vi "ECG_Monitor.vi"() -> ()   [LabVIEW 2011]
uses:
  <vilib>/Analysis/NI_AALBase.lvlib
  <vilib>/Analysis/3filter.llb/Butterworth Filter (DBL).vi
  <vilib>/Analysis/NI_AALPro.lvlib
  <vilib>/Analysis/2dsp.llb/Real FFT.vi
panel:
  out "Measured \nHeart Rate (bpm)":dbl
  in  "Set Threshold":i32(slide) scale=-600.0..600.0
  in  "start":bool
  in  "Save Data?":bool
  in  "High Cutoff Frequency (Hz)":i32
  in  "Filter Type":T1(ring)=enum."Band Pass"
  in  "Select Channel B":T2(ring)=enum."Zero"
  in  "Apply Filter?":bool
  in  "Low Cutoff Frequency (Hz)":i32=100
  out "Frequency Domain Signal":cluster{i32, dbl, "Power Spectrum":dbl[]}(graph)={0, 1.0, "Power Spectrum"=[]}
  out "Time Domain Signal":cluster{i32, dbl, dbl[]}(graph)={0, 1.0, []}
  in  "Select Channel A":enum16{"Channel 1", "Channel 2", "Channel 3"}(ring)
  out "Device Name":string="BioRadio 150"
  in  "Data Collection\nInterval (ms)":u32=1000
  in  "stop":bool
  out "DroppedPackets":u32
  out "BadPackets":u32
  out "GoodPackets":u32
  # "Transmission\nInformation"
  # "The signal observed below is given by (Channel A - Channel B)"
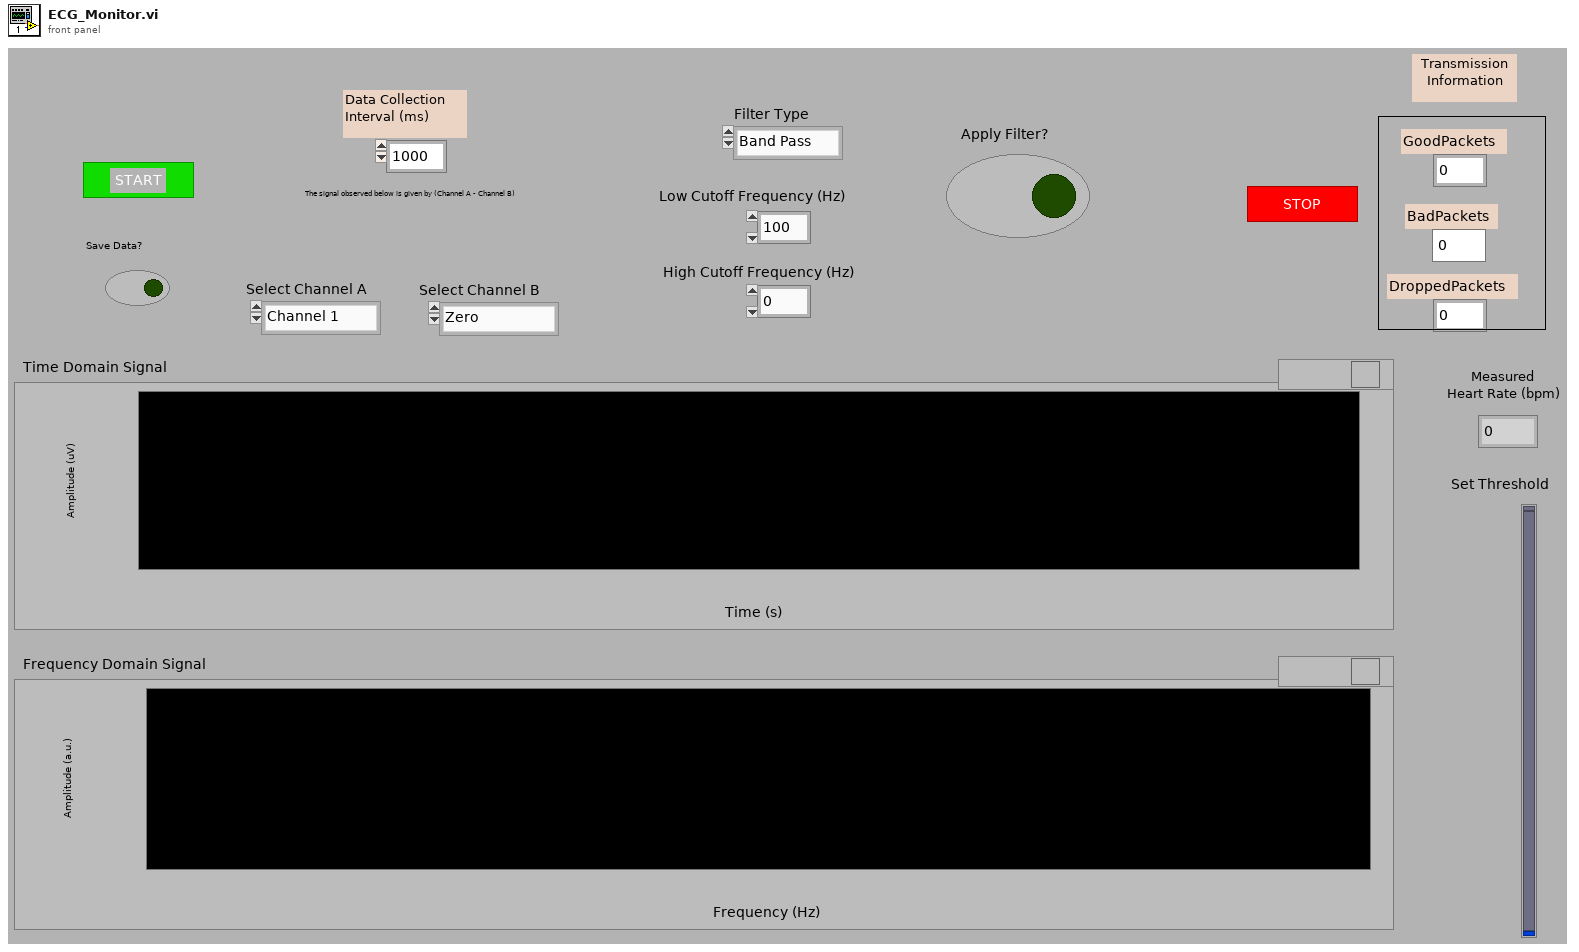
[diagram p1: front panel]
types:
  T1 = enum16{"Low Pass", "High Pass", "Band Pass", "Band Stop"}
  T2 = enum16{"Channel 1", "Channel 2", "Channel 3", "Zero"}
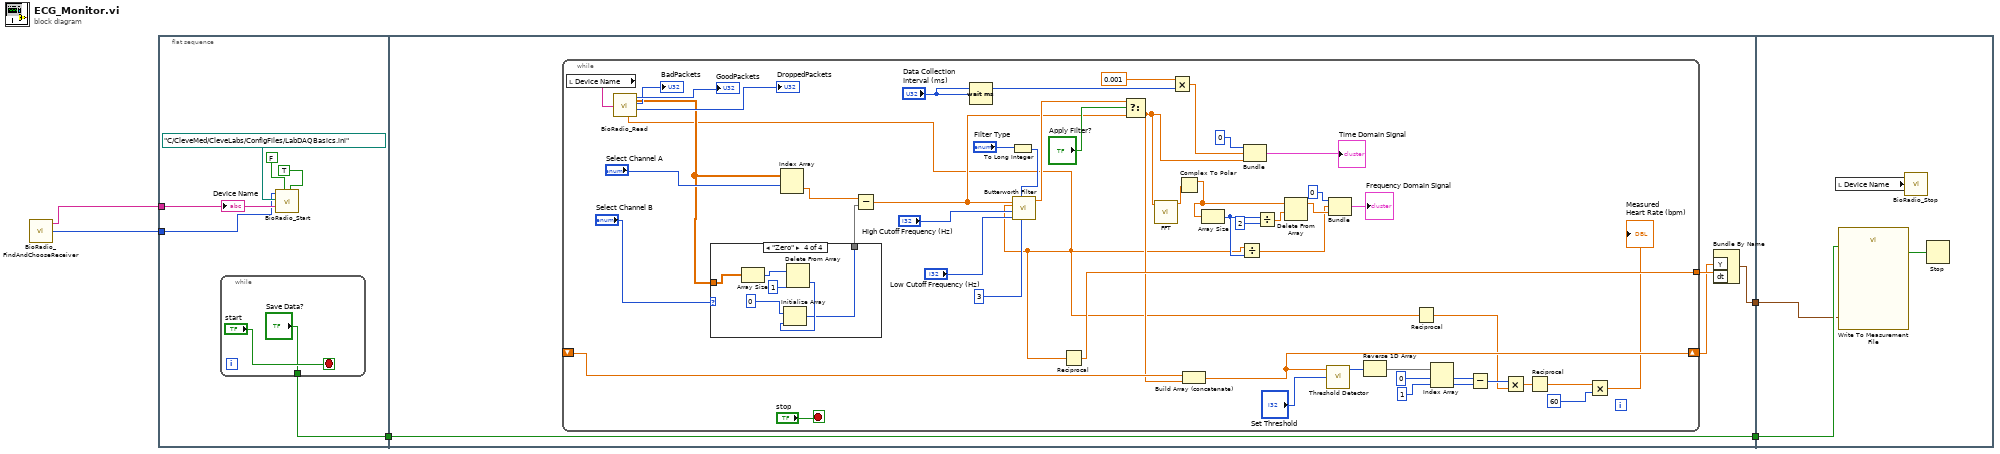
[diagram p0: block diagram]
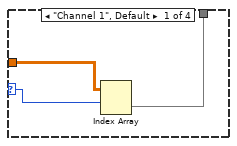
[diagram p2: hidden frame]
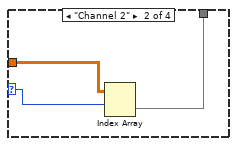
[diagram p3: hidden frame]
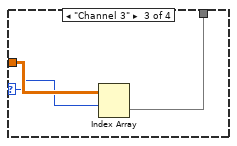
[diagram p4: hidden frame]
diagram:
  n1 = call "BioRadio_FindAndChooseReceiver.vi"() -> ("Device Name"=w2:string, "Port Number"=w1:i32)  [unwired: 2 out]
  n2 = flat-sequence {
    tunnel: [w8] -> w5
    tunnel: w2 -> [w7]
    tunnel: w1 -> [w6]
    tunnel: w5 -> [w17]
    tunnel: [w17] -> w4
    tunnel: [w14] -> w3
    tunnel: w4 -> [w85]
    tunnel: w3 -> [w83]
    frame #0 {
      n3 = while {
        tunnel: ["Save Data?"] -> w8
        stop <- "start" stop-if-true
      }
      n4 = call "BioRadio_Start.vi"("PingConfig"=TRUE, "ProgramDevice"=FALSE, "Device Name"=w7, "BioRadio ConfigFile Path"=path "C:/CleveMed/CleveLabs/ConfigFiles/LabDAQBasics.ini", "PortNum"=w6) -> ()  [unwired: 1 in, 6 out]
      "Device Name" <- w7
    }
    frame #1 {
      n5 = while {
        shift-right: [w33] -> w15
        shift-left: _ -> [w36]
        tunnel: [w35] -> w16
        stop <- "stop" stop-if-true
        n6 = local read "Device Name"() -> (w63:string)
        n7 = call "BioRadio_Read.vi"("Device Name"=w63) -> ("BioRadio Data"=w42:dbl[][], "Sample Rate"=w27:dbl, "GoodPackets"=→"GoodPackets":u32, "BadPackets"=→"BadPackets":u32, "DroppedPackets"=→"DroppedPackets":u32)  [unwired: 1 out]
        n8 = case shown="\"Zero\"" "Select Channel B" {
          selector: "Select Channel B" -> [w70 w73 w75 _]
          tunnel: w42 -> [w68 w72 w76 w81]
          tunnel: [w69 w71 w74 w77] -> w41
          frame "Channel 1", Default {
            n9 = Index Array(array=w68, index (row)=w70) -> (element=w69:dbl[])  [unwired: 1 in]
          }
          frame "Channel 2" {
            n10 = Index Array(array=w72, index (row)=w73) -> (element=w71:dbl[])  [unwired: 1 in]
          }
          frame "Channel 3" {
            n11 = Index Array(array=w76, index (row)=w75) -> (element=w74:dbl[])  [unwired: 1 in]
          }
          frame "Zero" {
            n12 = Array Size(array=w81) -> (size(s)=w80:i32[])
            n13 = Delete From Array(array=w80, index=1) -> (deleted portion=w78:i32)  [unwired: 1 in, 1 out]
            n14 = Initialize Array(0, w78) -> (w77:i32[])
          }
        }
        n15 = Index Array(array=w42, index (row)="Select Channel A") -> (element=w47:dbl[])  [unwired: 1 in]
        n16 = Subtract(x=w47, y=w41) -> (x-y=w46:dbl[])
        n17 = Wait (ms)(milliseconds to wait="Data Collection\nInterval (ms)") -> ()  [unwired: 1 out]
        n18 = To Long Integer(number="Filter Type") -> (32bit integer=w39:i32)
        n19 = call-poly <vilib>:"Butterworth Filter.vi"("order"=3, "filter type"=w39, "low cutoff freq: fl"="Low Cutoff Frequency (Hz)", "high cutoff freq: fh"="High Cutoff Frequency (Hz)", "sampling freq: fs"=w27, "X"=w46) -> ("Filtered X"=w58:dbl[])  [unwired: 1 in, 2 out]
        n20 = Reciprocal(x=w27) -> (1/x=w35:dbl)
        n21 = Select(t=w58, s="Apply Filter?", f=w46) -> (s? t:f=w34:dbl[])
        n22 = call-poly <vilib>:"FFT.vi"("X"=w34) -> ("FFT {X}"=w45:cdb[])  [unwired: 2 in, 8 out]
        n23 = Multiply(x=0.001, y="Data Collection\nInterval (ms)") -> (x*y=w28:dbl)
        n24 = Complex To Polar(r * e^(i*theta)=w45) -> (r=w44:dbl[])  [unwired: 1 out]
        n25 = Build Array (concatenate)(w36, w34) -> (w33:dbl[])
        n26 = Array Size(array=w44) -> (size(s)=w51:i32)
        n27 = Divide(x=w27, y=w51) -> (x/y=w50:dbl)
        n28 = Bundle(0, w28, "Filtered X"=w34) -> (→"Time Domain Signal":cluster{i32, dbl, "Filtered X":dbl[]})  [unwired: 1 out]
        n29 = Divide(x=w51, y=2) -> (x/y=w54:dbl)
        n30 = Delete From Array(array=w44, length=w54) -> (array with subset deleted=w53:dbl[])  [unwired: 1 in, 1 out]
        n31 = call <vilib>:"Threshold Detector.vi"("threshold"="Set Threshold", "X"=w33) -> ("Indices"=w22:i32[])  [unwired: 1 in, 2 out]
        n32 = Bundle(0, w50, w53) -> (→"Frequency Domain Signal":cluster{i32, dbl, dbl[]})  [unwired: 1 out]
        n33 = Reverse 1D Array(array=w22) -> (reversed array=w21:i32[])
        n34 = Reciprocal(x=w27) -> (1/x=w26:dbl)
        n35 = Index Array(array=w21, index #1=0, index #2=1) -> (element #1=w31:i32, element #2=w30:i32)
        n36 = Subtract(x=w31, y=w30) -> (x-y=w29:i32)
        n37 = Multiply(x=w29, y=w26) -> (x*y=w18:dbl)
        n38 = Reciprocal(x=w18) -> (1/x=w24:dbl)
        n39 = Multiply(x=w24, y=60) -> (x*y=→"Measured \nHeart Rate (bpm)":dbl)
      }
      n40 = Bundle By Name("Y"=w15, "dt"=w16) -> (w14:waveform(dbl))  [unwired: 1 out]
    }
    frame #2 {
      n41 = local read "Device Name"() -> (w86:string)
      n42 = call "Write To Measurement File"("Signals"=w83, "Enable"=w85) -> ("Saving Data"=w84:bool)  [unwired: 5 in, 12 out]
      n43 = call "BioRadio_Stop.vi"("Device Name"=w86) -> ()  [unwired: 1 out]
      n44 = Stop(stop? (T)=w84) -> ()
    }
  }
